vi "SDCP BTR Test.vi"() -> ()   [LabVIEW 2020]
uses:
  Typedefs/SDCP BTR Params.ctl
  Typedefs/SDCP BTR Parameter cluster.ctl
  Typedefs/SDCP BTR Parameter data type.ctl
  Typedefs/SDCP - Serial Port Control - Commands.ctl
panel:
  out "Read BTR parameters":T1[](array[typedef])
  in  "BTR Parameter File Path":path=path "E:/Projects/System Diagnostics and Control Protocol/SDCP_LabVIEW/Parameter Files/test.btp"
  in  "Number of transfers":u16=10
  in  "Parameter IDs":u8[](array[numeric])=[8, 9, 10, 11]
  out "BTR status":T3
  in  "Baud rate":u32=115200
  in  "COM Port":refnum<visa-resource-name>="COM5"
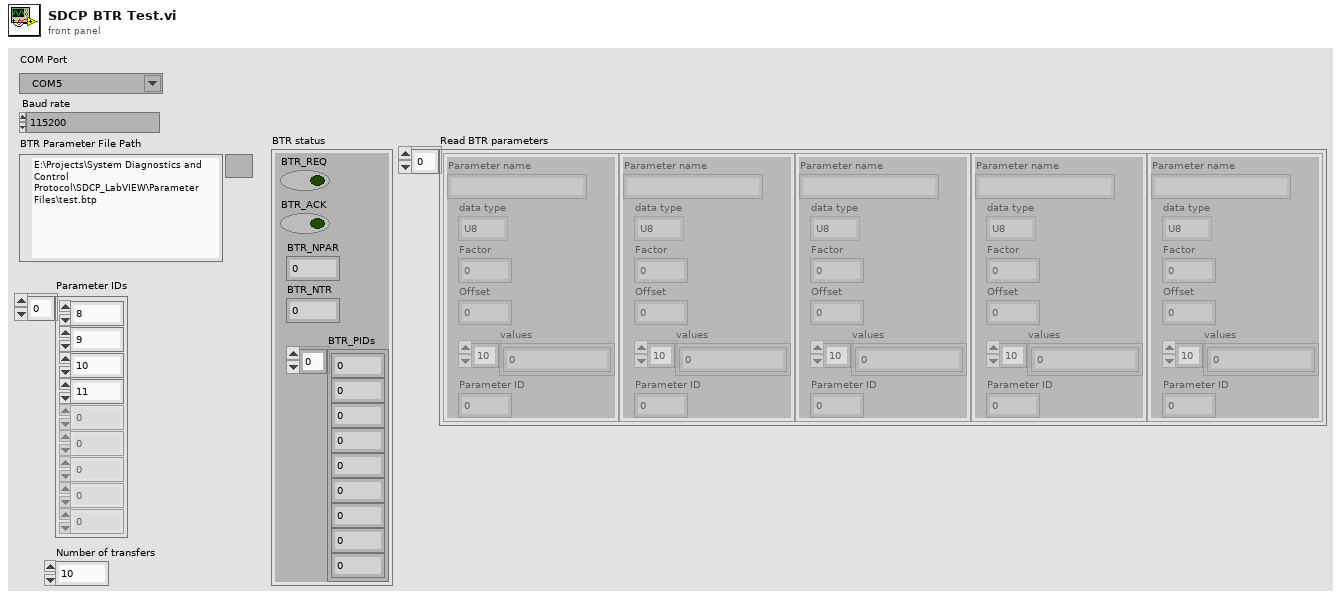
[diagram p1: front panel]
types:
  T1 = typedef "SDCP BTR Parameter cluster.ctl" = cluster{"Parameter name":string, "data type":T2, "Factor":dbl, "Offset":dbl, "values":dbl[], "Parameter ID":i32}
  T2 = typedef "SDCP BTR Parameter data type.ctl" = enum16{"U8", "I8", "U16", "I16", "U32", "I32", "F32"}
  T3 = typedef "SDCP BTR Params.ctl" = cluster{"BTR_REQ":bool, "BTR_ACK":bool, "BTR_NPAR":i32, "BTR_NTR":i32, "BTR_PIDs":u8[]}
  T4 = typedef "SDCP - Serial Port Control - Commands.ctl" = enum16{"Open", "Read", "Write", "Get instance", "Close"}
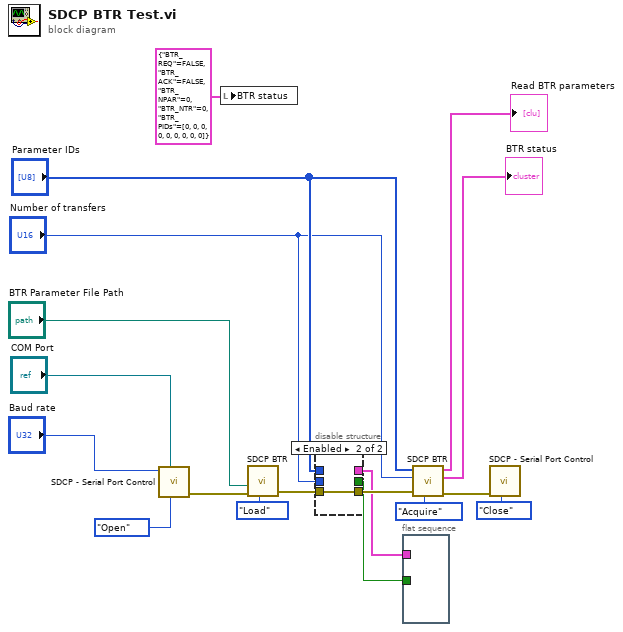
[diagram p0: block diagram]
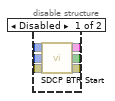
[diagram p2: hidden frame]
diagram:
  n1 = call "SDCP - Serial Port Control.vi"("Command"=SDCP_-_Serial_Port_Control_-_Commands."Open", "VISA resource name"="COM Port", "Baud rate"="Baud rate") -> ("error out"=w14:errorcluster)  [unwired: 5 in, 3 out]
  n2 = local write "BTR status"(T3 {"BTR_REQ"=FALSE, "BTR_ACK"=FALSE, "BTR_NPAR"=0, "BTR_NTR"=0, "BTR_PIDs"=[0, 0, 0, 0, 0, 0, 0, 0, 0]} ("BTR status")) -> ()
  n3 = call "SDCP BTR.vi"("Command"=enum16{"Load", "Acquire"}."Load", "error in (no error)"=w14, "Block transfer parameters file path"="BTR Parameter File Path") -> ("error out"=w7:errorcluster)  [unwired: 5 in, 3 out]
  n4 = disable-structure shown="Enabled" {
    disable-tunnel: w7 -> [w24 w25]
    disable-tunnel: [w23 w25] -> w6
    disable-tunnel: "Parameter IDs" -> [w22 _]
    disable-tunnel: "Number of transfers" -> [w21 _]
    disable-tunnel: [w20 _] -> w3
    disable-tunnel: [w19 _] -> w2
    frame Disabled {
      n5 = call "SDCP BTR Start.vi"("error in (no error)"=w24, "Number of transfers"=w21, "Parameter IDs"=w22) -> ("error out"=w23:errorcluster, "No timeout"=w19:bool, "out"=w20:T3)
    }
    frame Enabled {
    }
  }
  n6 = flat-sequence {
    tunnel: w3 -> [_]
    tunnel: w2 -> [_]
    frame #0 {
    }
  }
  n7 = call "SDCP BTR.vi"("Command"=enum16{"Load", "Acquire"}."Acquire", "error in (no error)"=w6, "Number of transfers"="Number of transfers", "Parameter IDs"="Parameter IDs") -> ("error out"=w10:errorcluster, "Status"=→"BTR status":T3, "Read BTR parameters"=→"Read BTR parameters":T1[])  [unwired: 4 in, 1 out]
  n8 = call "SDCP - Serial Port Control.vi"("Command"=SDCP_-_Serial_Port_Control_-_Commands."Close", "error in (no error)"=w10) -> ()  [unwired: 6 in, 4 out]
